vi "flash.vi"   [LabVIEW 2015]
uses:
  <vilib>/rvi/Emulation/niFpgaGetClockAttributes.vi
  <vilib>/rvi/Emulation/niFpgaSctlEmulationGetInTimedLoop.vi
  <vilib>/rvi/Emulation/niFpgaEmulationReportErrorSimple.vi
  <vilib>/rvi/eio/common/nirviEmuTemplateMethod_errors.vi
  <vilib>/rvi/Emulation/niFpgaCriticalErrorInLSC.vi
  <vilib>/eio/EIONode/EIONode.xnode
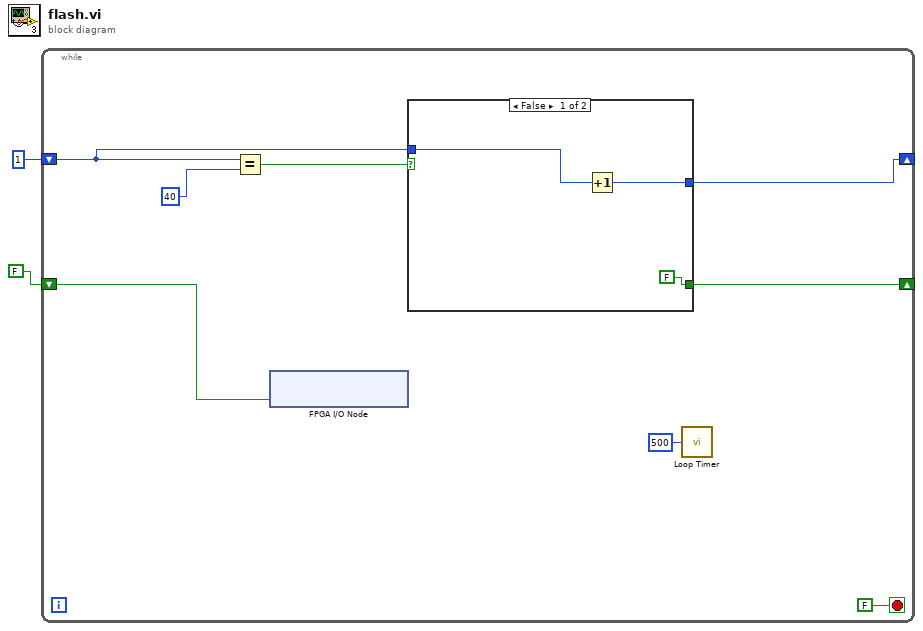
[diagram p0: block diagram]
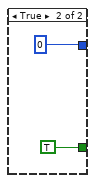
[diagram p2: hidden frame]
diagram:
  n1 = while {
    shift-right: [w4] -> _
    shift-left: FALSE -> [w9]
    shift-right: [w5] -> _
    shift-left: i16 1 -> [w6]
    stop <- FALSE stop-if-true
    n2 = Equal?(x=w6, y=i16 40) -> (x = y?=w7:bool)
    n3 = xnode "FPGA I/O Node"("ConnectorC/DIO4"=w9) -> ()  [unwired: 1 in, 1 out]
    n4 = case shown="False" w7 {
      tunnel: w6 -> [w13 _]
      tunnel: [w12 i16 0] -> w5
      tunnel: [FALSE TRUE] -> w4
      frame False {
        n5 = Increment(x=w13) -> (x+1=w12:i16)
      }
      frame True {
      }
    }
    n6 = call "Loop Timer"("Count(mSec)"=u32 500) -> ()  [unwired: 1 out]
  }
